vi "Queue_LV2.vi"(5 "element in":T1, 11 "error in (no error)":errorcluster, 13 "Operation":T2) -> (6 "element out":T1, 15 "error IO":errorcluster)   [LabVIEW 2023, in "task_1.lvlib"]
doc: "Add and pop element from the queue."
uses:
  task_1.lvlib
  Controls/Queue_op.ctl
  Data_TC.ctl
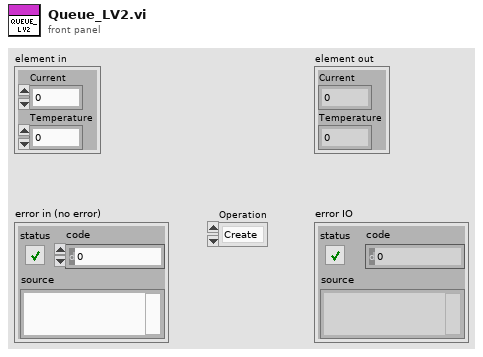
[diagram p1: front panel]
types:
  T1 = typedef "task_1.lvlib/Data_TC.ctl" = cluster{"Current":dbl, "Temperature":dbl}
  T2 = typedef "task_1.lvlib/Queue_op.ctl" = enum16{"Create", "Enqueue", "Dequeue", "Destroy"}
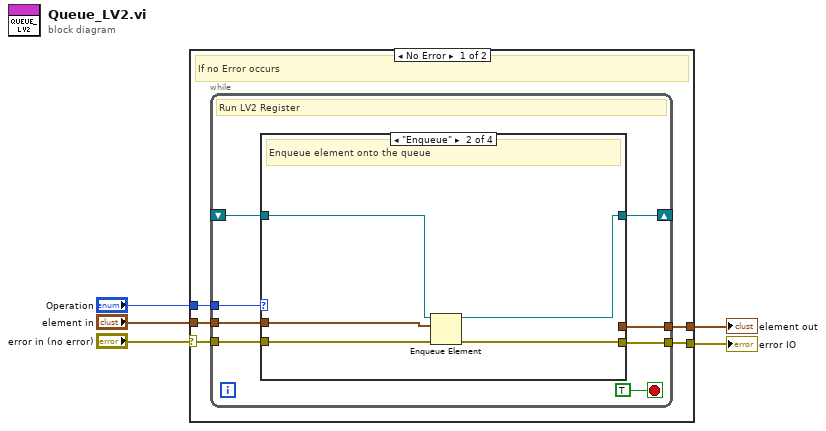
[diagram p0: block diagram]
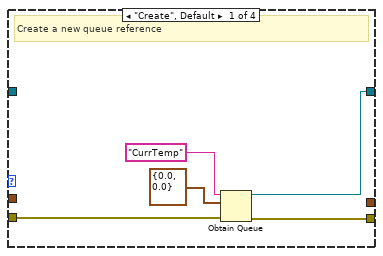
[diagram p2: hidden frame]
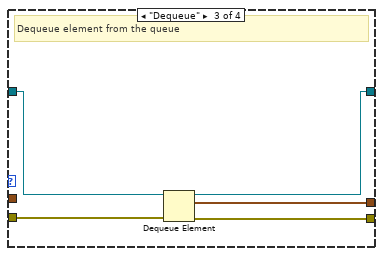
[diagram p3: hidden frame]
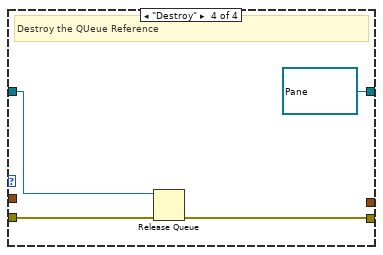
[diagram p4: hidden frame]
diagram:
  n1 = case shown="No Error" "error in (no error)" {
    selector: "error in (no error)" -> [w9 w38]
    tunnel: "Operation" -> [w10 _]
    tunnel: [w8 w38] -> w1
    tunnel: "element in" -> [w7 _]
    tunnel: [w6 _] -> w2
    frame No Error {
      # "If no Error occurs"
      n2 = while {
        tunnel: w10 -> [w18]
        tunnel: w9 -> [w17]
        tunnel: [w16] -> w8
        shift-right: [w15] -> _
        shift-left: _ -> [w14]
        tunnel: w7 -> [w13]
        tunnel: [w11] -> w6
        stop <- TRUE stop-if-true
        # "Run LV2 Register"
        n3 = case shown="\"Enqueue\"" w18 {
          tunnel: w17 -> [w21 w28 w33 w37]
          tunnel: [w20 w27 w32 w36] -> w16
          tunnel: [w19 w24 w30 refnum<queue> refnum ("queue out")] -> w15
          tunnel: w14 -> [_ w26 w31 w35]
          tunnel: w13 -> [_ w25 _ _]
          tunnel: [_ _ w29 _] -> w11
          frame "Create", Default {
            # "Create a new queue reference"
            n4 = Obtain Queue(name (unnamed)="CurrTemp", element data type=T1 {"Current"=0.0, "Temperature"=0.0}, error in (no error)=w21) -> (queue out=w19:refnum<queue>, error out=w20:errorcluster)  [unwired: 2 in, 1 out]
          }
          frame "Enqueue" {
            # "Enqueue element onto the queue"
            n5 = Enqueue Element(queue=w26, element=w25, error in (no error)=w28) -> (queue out=w24:refnum<queue>, error out=w27:errorcluster)  [unwired: 1 in, 1 out]
          }
          frame "Dequeue" {
            # "Dequeue element from the queue"
            n6 = Dequeue Element(queue=w31, error in (no error)=w33) -> (queue out=w30:refnum<queue>, element=w29:T1, error out=w32:errorcluster)  [unwired: 1 in, 1 out]
          }
          frame "Destroy" {
            # "Destroy the QUeue Reference"
            n7 = Release Queue(queue=w35, error in (no error)=w37) -> (error out=w36:errorcluster)  [unwired: 1 in, 2 out]
          }
        }
      }
    }
    frame Error {
      # "If error occurs"
    }
  }
  "element out" <- w2
  "error IO" <- w1
